vi "Set_Parameter_Instrument (Json).vi"(8 "error in (no error)":errorcluster caption="entrée d'erreur (pas d'erreur)", 10 "Parameter (Json)":string, 11 "Delay en entrée":refnum<class "P2056_Provisionning.lvclass">) -> (0 "error out":errorcluster caption="sortie d'erreur", 3 "Delay en sortie":refnum<class "P2056_Provisionning.lvclass">)   [LabVIEW 2020, in "Library Test.lvlib" / "P2056_Provisionning.lvclass"]
uses:
  P2056_Provisionning.lvclass
  C:/Users/ngarcin/OneDrive - Altyor/Standard TB/Class/Test/Test (Default)/Test (Default).lvclass
  Test_Without_Instr/Test_Without_Inst.lvclass
  P2056_Provisionning.lvclass/P2056_Provisionning.ctl
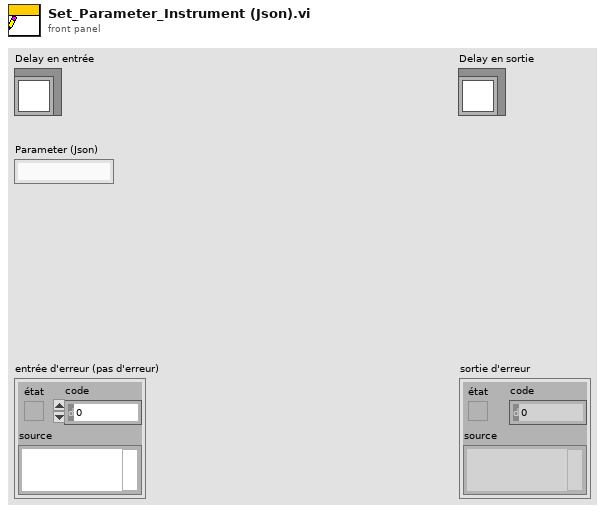
[diagram p1: front panel]
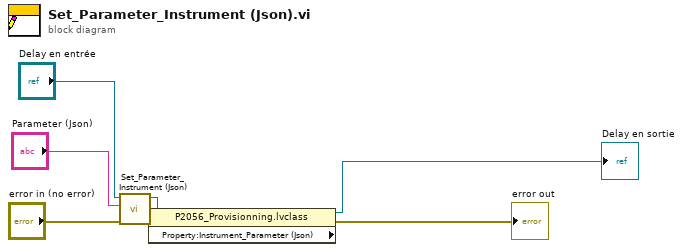
[diagram p0: block diagram]
diagram:
  n1 = call-parent "Set_Parameter_Instrument (Json).vi"("error in (no error)"="error in (no error)", "Parameter (Json)"="Parameter (Json)", "Test (Default) en entrée"="Delay en entrée") -> ("error out"=w3:errorcluster, "Test (Default) en sortie"=w4:refnum<class "P2056_Provisionning.lvclass">)  [unwired: 7 in]
  n2 = property class="P2056_Provisionning.lvclass" props=["Property:Instrument_Parameter (Json)"](reference=w4, error in=w3) -> (reference out=→"Delay en sortie":refnum<class "P2056_Provisionning.lvclass">, error out=→"error out":errorcluster)  [unwired: 1 out]
